vi "Cast Command to Transfer Group.vi"(8 "error in (no error)":errorcluster, 10 "command parameters":T1, 11 "Plugin Thread in":refnum<class "Plugin Thread.lvclass">) -> (0 "error out":errorcluster, 1 "Transfer Group iteration":u64, 2 "Transfer Group id":i32, 3 "Plugin Thread out":refnum<class "Plugin Thread.lvclass">)   [LabVIEW 2017, in "DSF Core.lvlib" / "Plugin Thread.lvclass"]
uses:
  Thread/Plugin/Plugin Thread.lvclass
  Interface/Plugin/Command Parameters.ctl
  Interface/Plugin/Plugin Interface.lvclass
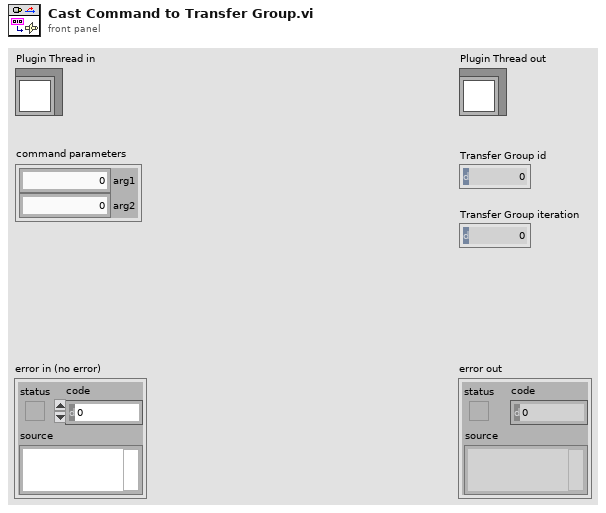
[diagram p1: front panel]
types:
  T1 = typedef "DSF Core.lvlib/Plugin Interface.lvclass/Command Parameters.ctl" = cluster{"arg1":u64, "arg2":u64}
  T2 = cluster{"Transfer Group ID":i32, "unused":i32, "Transfer Group iteration":u64}
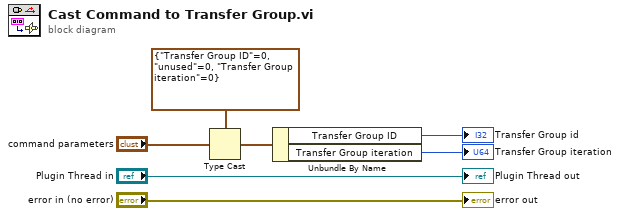
[diagram p0: block diagram]
diagram:
  n1 = Type Cast(type=T2 {"Transfer Group ID"=0, "unused"=0, "Transfer Group iteration"=0}, x="command parameters") -> (*(type *) &x=w5:T2)
  n2 = Unbundle By Name(w5) -> ("Transfer Group ID"=→"Transfer Group id":i32, "Transfer Group iteration"=→"Transfer Group iteration":u64)
  "error out" <- "error in (no error)"
  "Plugin Thread out" <- "Plugin Thread in"
